vi "ZAlign_ConPanePos.vi"(4 "Grid_Size":i16, 6 "ScaledGridSize":i16, 9 "Positions":u32[](array[numeric]), 10 "Max right location":u32, 11 "Height":u32) -> (1 "Positions-Grid":u32[](array[numeric]), 2 "Height+Grid":u32, 3 "Positions+Grid+MaxRight":u32[](array[numeric]))   [LabVIEW 2014, in "ZAlign.lvlib"]
doc: "ZAlign.lvlib:ZAlign_ConPanePos.vi\n----------------------------------------------\nConectorPane Rahmen berechnen.\n\nInputs:\n---------------------\n- Grid_Size : I16; \n- ScaledGridSize : I16; \n- Positions : 1DArrayOfU32; \n- Max right location : U32; \n- Height : U32; \n\nOutputs:\n---------------------\n- Positions-Grid : 1DArrayOfU32; \n- Height+Grid : U32; \n- Positions+Grid+MaxRight : 1DArrayOfU32; \n\n----------------------------------------------\n26.03.2015 jcm\nZühlke Engineering AG\nCH-8952 Schlieren\nwww.zuehlke.com"
uses:
  ZAlign.lvlib
panel:
  # "Connector Pane"
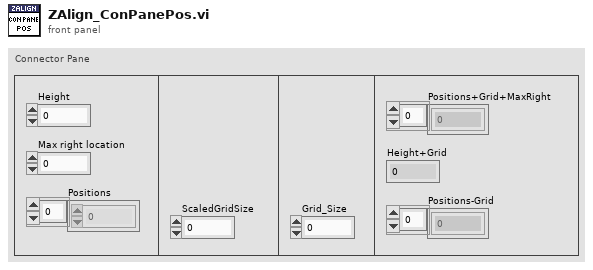
[diagram p1: front panel]
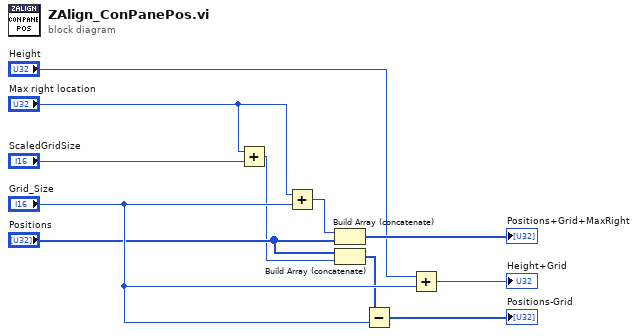
[diagram p0: block diagram]
diagram:
  n1 = Add(x="Max right location", y="ScaledGridSize") -> (x+y=w2:u32)
  n2 = Add(x="Max right location", y="Grid_Size") -> (x+y=w7:u32)
  n3 = Build Array (concatenate)(w7, "Positions") -> (→"Positions+Grid+MaxRight":u32[])
  n4 = Build Array (concatenate)("Positions", w2) -> (w8:u32[])
  n5 = Subtract(x=w8, y="Grid_Size") -> (x-y=→"Positions-Grid":u32[])
  n6 = Add(x="Height", y="Grid_Size") -> (x+y=→"Height+Grid":u32)
